vi "Run Tx - Handle Port Tx Check.vi"(8 "error in (no error)":errorcluster, 10 "Destination Port":u16, 11 "Port as Channel":bool) -> (0 "error out":errorcluster, 3 "Transmit?":bool)   [LabVIEW 2021, in "UDP-Custom-Device Engine.lvlib"]
uses:
  UDP-Custom-Device Engine.lvlib
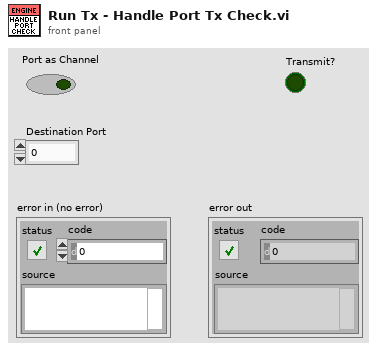
[diagram p1: front panel]
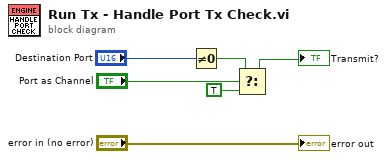
[diagram p0: block diagram]
diagram:
  n1 = Not Equal To 0?(x="Destination Port") -> (x != 0?=w4:bool)
  n2 = Select(t=w4, s="Port as Channel", f=TRUE) -> (s? t:f=→"Transmit?":bool)
  "error out" <- "error in (no error)"
